vi "pmu_Get Buffer Size.vi"(8 "error in (no error)":errorcluster, 9 "PMU System Info in":refnum<class "PMU System Info.lvclass">, 11 "physical channels":T1[](array[typedef])) -> (0 "error out":errorcluster, 1 "PMU System Info out":refnum<class "PMU System Info.lvclass">, 3 "buffer size (samples)":u32=250)   [LabVIEW 2013, in "NI_EP_PMU.lvlib"]
doc: "This VI determines size of circular buffer which hold data read from DMA FIFO. The buffer must be large enough to hold sufficient data for both frequency and phasor evaluation window."
uses:
  <vilib>/addons/Electrical Power/PMU/NI_EP_PMU.lvlib
  <vilib>/addons/Electrical Power/PMU/Common/Classes/PMU System Info/PMU System Info.lvclass
  <vilib>/addons/Electrical Power/PMU/Common/Controls/pmu_Physical Channel.ctl
  <vilib>/addons/Electrical Power/PMU/Common/Controls/pmu_Channel Phase.ctl
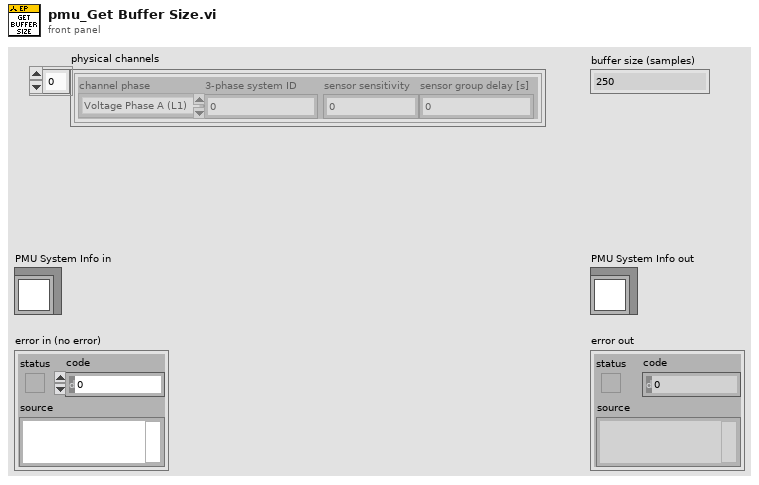
[diagram p1: front panel]
types:
  T1 = typedef "NI_EP_PMU.lvlib/pmu_Physical Channel.ctl" = cluster{"channel phase":T2, "3-phase system ID":u8, "sensor sensitivity":dbl, "sensor group delay [s]":dbl}
  T2 = typedef "NI_EP_PMU.lvlib/pmu_Channel Phase.ctl" = enum16{"Voltage Phase A (L1)", "Voltage Phase B (L2)", "Voltage Phase C (L3)", "Voltage Phase N (Neutral)", "Current Phase A (L1)", "Current Phase B (L2)", "Current Phase C (L3)", "Current Phase N (Neutral)"}
  T3 = typedef "NI_EP_PMU.lvlib/pmu_CFG Class.ctl" = cluster{"station name":string, "PMU ID":u16, "time base":u32, "nominal frequency":enum16{"50 Hz", "60 Hz"}, "reporting rate":i16, "phasor number":u16, "analog number":u16, "digital number":u16, "channel names":string[], "phasor units":u32[], "analog units":u32[], "digital units":u32[], "data format":u16, "number of PMUs":u16}
  T4 = typedef "NI_EP_PMU.lvlib/pmu_ROCOF Detector Settings.ctl" = cluster{"ROCOF window width":i32}
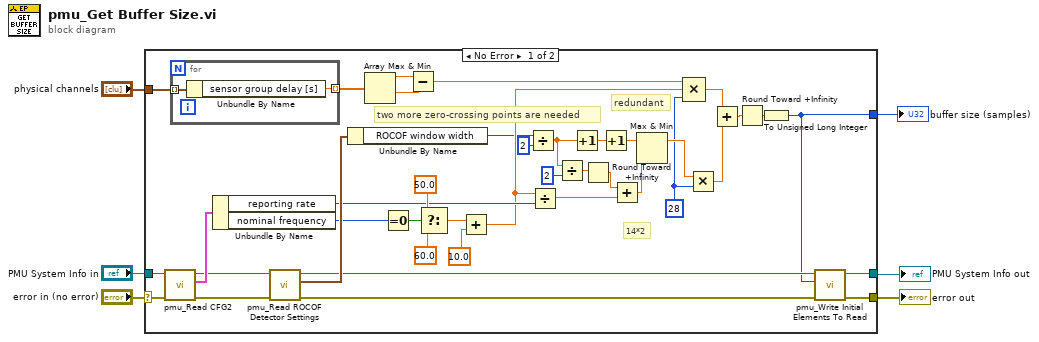
[diagram p0: block diagram]
diagram:
  n1 = case shown="No Error" "error in (no error)" {
    selector: "error in (no error)" -> [w45 w49]
    tunnel: [w23 w49] -> w6
    tunnel: "PMU System Info in" -> [w46 w50]
    tunnel: [w22 w50] -> w4
    tunnel: [w19 _] -> w2
    tunnel: "physical channels" -> [w35 _]
    frame No Error {
      w25 = 28 ("y")
      # "two more zero-crossing points are needed"
      # "redundant"
      # "14*2"
      n2 = call <vilib>:"pmu_Read CFG2.vi"("error in (no error)"=w45, "system info in"=w46) -> ("error out"=w17:errorcluster, "CFG-2"=w41:T3, "system info out"=w18:refnum<class "PMU System Info.lvclass">)  [unwired: 7 in]
      n3 = for {
        tunnel: w35 -> [w48] mode=indexing
        tunnel: [w47] -> w34 mode=indexing
        n4 = Unbundle By Name(w48) -> ("sensor group delay [s]"=w47:dbl)
      }
      n5 = Unbundle By Name(w41) -> ("reporting rate"=w31:i16, "nominal frequency"=w39:enum16{"50 Hz", "60 Hz"})
      n6 = call <vilib>:"pmu_Read ROCOF Detector Settings.vi"("error in (no error)"=w17, "system info in"=w18) -> ("error out"=w20:errorcluster, "ROCOF detector settings"=w44:T4, "system info out"=w21:refnum<class "PMU System Info.lvclass">)  [unwired: 7 in]
      n7 = Unbundle By Name(w44) -> ("ROCOF window width"=w7:i32)
      n8 = Array Max & Min(array=w34) -> (max value=w33:dbl, min value=w32:dbl)  [unwired: 2 out]
      n9 = Equal To 0?(x=w39) -> (x = 0?=w40:bool)
      n10 = Subtract(x=w33, y=w32) -> (x-y=w27:dbl)
      n11 = Select(t=50.0, s=w40, f=60.0) -> (s? t:f=w28:dbl)
      n12 = Add(x=w28, y=10.0) -> (x+y=w26:dbl)
      n13 = Divide(x=w7, y=2) -> (x/y=w9:dbl)
      n14 = Divide(x=w26, y=w31) -> (x/y=w15:dbl)
      n15 = Divide(x=w9, y=2) -> (x/y=w12:dbl)
      n16 = Increment(x=w9) -> (x+1=w10:dbl)
      n17 = Round Toward +Infinity(x=w12) -> (ceil(x): smallest int >= x=w11:dbl)
      n18 = Increment(x=w10) -> (x+1=w8:dbl)
      n19 = Add(x=w11, y=w15) -> (x+y=w14:dbl)
      n20 = Max & Min(x=w8, y=w14) -> (max(x,y)=w30:dbl)  [unwired: 1 out]
      n21 = Compound Arithmetic op=MULTIPLY(w27, w26, w25) -> (w24:dbl)
      n22 = Multiply(x=w30, y=w25) -> (x*y=w29:dbl)
      n23 = Add(x=w29, y=w24) -> (x+y=w42:dbl)
      n24 = Round Toward +Infinity(x=w42) -> (ceil(x): smallest int >= x=w43:dbl)
      n25 = To Unsigned Long Integer(number=w43) -> (unsigned 32bit integer=w19:u32)
      n26 = call <vilib>:"pmu_Write Initial Elements To Read.vi"("error in (no error)"=w20, "initial elements to read"=w19, "system info in"=w21) -> ("error out"=w23:errorcluster, "system info out"=w22:refnum<class "PMU System Info.lvclass">)  [unwired: 7 in]
    }
    frame Error {
    }
  }
  "error out" <- w6
  "buffer size (samples)" <- w2
  "PMU System Info out" <- w4
